vi "AT Queue Buffer A.vi"(8 "error in (no error)":errorcluster, 9 "PtrSize":i64, 10 "Ptr":u64, 11 "Handle":i32) -> (0 "error out":errorcluster, 3 "Status":i32)   [LabVIEW 2019]
doc: "Queue Buffer\n\nOutput:\n I32 Status\n\nInput:\n I32 Handle\n U32 Ptr\n I64 PtrSize\n\nThis function configures the area of memory into which acquired images will be stored. You can call this\nfunction multiple times to set up storage for consecutive images in a series. The order in which buffers are\nqueued is the order in which they will be used on a first in, first out (FIFO) basis. The PtrSize parameter should be equal to the size of an individual image in number of bytes. This function may be called before the acquisition starts, after the acquisition starts or a combination of the two. Any buffers queued using this function should not be modified or deallocated by the calling application until they are either returned from the WaitBuffer function, or the Flush function is called."
uses:
  atcoreA.dll
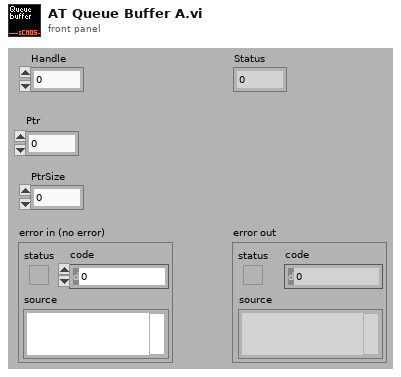
[diagram p1: front panel]
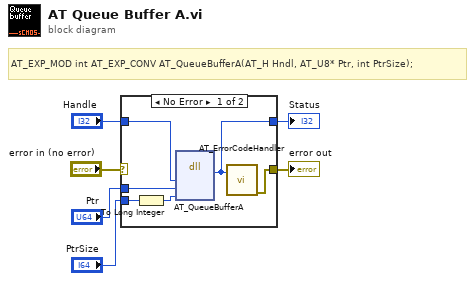
[diagram p0: block diagram]
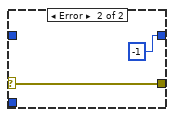
[diagram p2: hidden frame]
diagram:
  # "AT_EXP_MOD int AT_EXP_CONV AT_QueueBufferA(AT_H Hndl, AT_U8* Ptr, int PtrSize);"
  n1 = case shown="No Error" "error in (no error)" {
    selector: "error in (no error)" -> [_ w14]
    tunnel: [w7 -1 ("return type")] -> w6
    tunnel: "Handle" -> [w12 _]
    tunnel: "Ptr" -> [w11 _]
    tunnel: "PtrSize" -> [w10 _]
    tunnel: [w8 w14] -> w1
    frame No Error {
      n2 = To Long Integer(number=w10) -> (32bit integer=w9:i32)
      n3 = dll-call lib="atcoreA.dll" fn="AT_QueueBufferA"("Handle"=w12, "Ptr"=w11, "PtrSize"=w9) -> ("Status"=w7:i32)  [unwired: 6 in, 2 out]
      n4 = call <userlib>:"AT_ErrorCodeHandler.vi"("Error"=w7) -> ("error out"=w8:errorcluster)  [unwired: 6 in]
    }
    frame Error {
    }
  }
  "Status" <- w6
  "error out" <- w1
